vi "test4-ArgumentCanBeTakenToTargetModule.vi"(8 "error in (no error)":errorcluster, 11 "TestCase in":refnum<class "testcase-CSMArgument.lvclass">) -> (0 "error out":errorcluster, 3 "TestCase out":refnum<class "testcase-CSMArgument.lvclass">)   [LabVIEW 2017, in "testcase-CSMArgument.lvclass"]
uses:
  testcase-CSMArgument.lvclass
  a780a543-d55d-4312-9572-3fc81e4783fb.vi
  <vilib>/addons/_JKI Toolkits/VI Tester/TestCase.llb/TestCase.lvclass
  src/user.lib/_NEVSTOP/Communicable State Machine(CSM)/Communicable State Machine.lvlib
  CSM/CSM-Testcase.lvlib
  C:/Program Files (x86)/National Instruments/LabVIEW 2017/vi.lib/addons/_JKI Toolkits/VI Tester/TestCase.llb/TestCase.lvclass
panel:
  out "LoopCount":i32
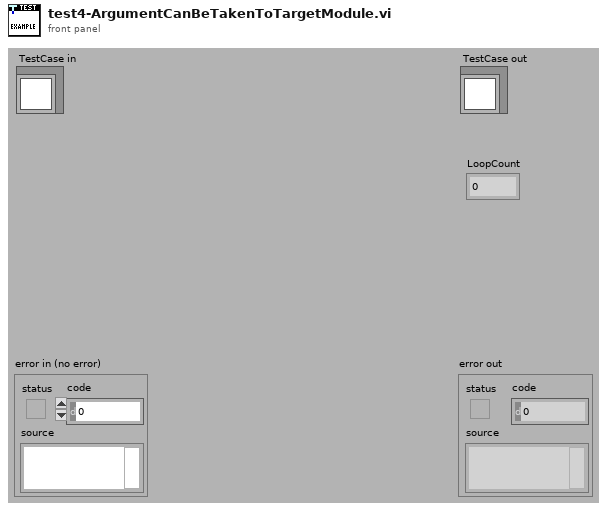
[diagram p1: front panel]
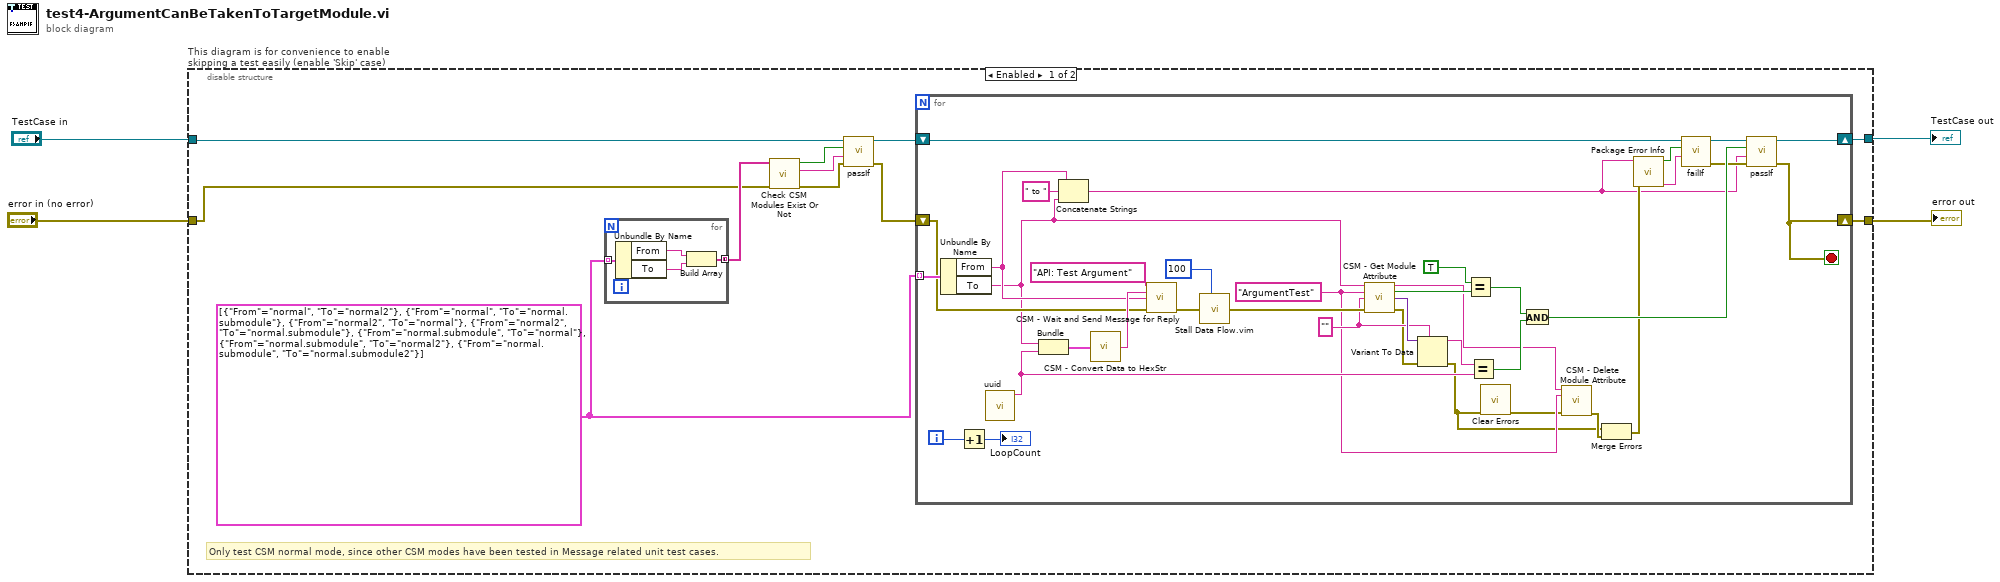
[diagram p0: block diagram]
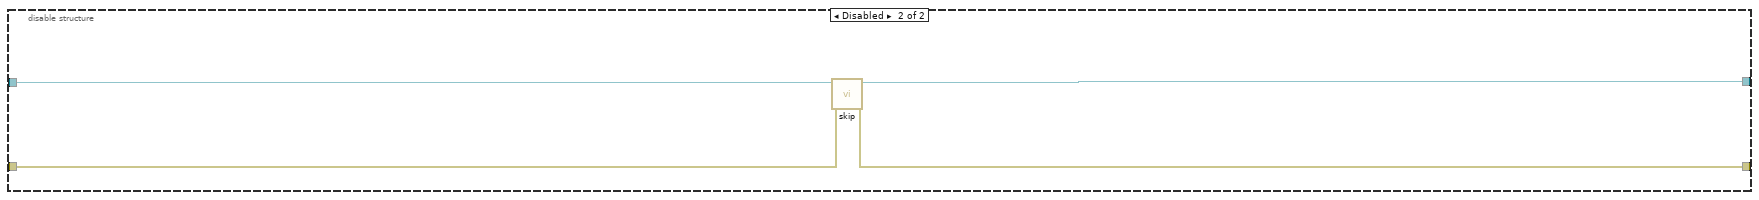
[diagram p2: hidden frame]
diagram:
  n1 = disable-structure "This diagram is for convenience to enable skipping a test easily (enable 'Skip' case)" shown="Enabled" {
    disable-tunnel: "TestCase in" -> [w8 w60]
    disable-tunnel: [w15 w58] -> w1
    disable-tunnel: [w14 w59] -> w3
    disable-tunnel: "error in (no error)" -> [w6 w57]
    frame Enabled {
      w9 = cluster{"From":string, "To":string}[] [{"From"="normal", "To"="normal2"}, {"From"="normal", "To"="normal.submodule"}, {"From"="normal2", "To"="normal"}, {"From"="normal2", "To"="normal.submodule"}, {"From"="normal.submodule", "To"="normal"}, {"From"="normal.submodule", "To"="normal2"}, {"From"="normal.submodule", "To"="normal.submodule2"}]
      # "Only test CSM normal mode, since other CSM modes have been tested in Message related unit test cases."
      n2 = for {
        tunnel: w9 -> [w19] mode=indexing
        tunnel: [w16] -> w12 mode=concatenating
        n3 = Unbundle By Name(w19) -> ("From"=w18:string, "To"=w17:string)
        n4 = Build Array(w18, w17) -> (w16:string[])
      }
      n5 = call "Check CSM Modules Exist Or Not.vi"("error in"=w6, "CSM names in"=w12) -> ("error out"=w10:errorcluster, "Debug string"=w11:string, "All Modules Exist?"=w13:bool)  [unwired: 7 in]
      n6 = call-dynamic "passIf.vi"("error in (no error)"=w10, "message (\"\")"=w11, "pass"=w13, "TestCase in"=w8) -> ("error out"=w5:errorcluster, "TestCase out"=w7:refnum<class "testcase-CSMArgument.lvclass">)  [unwired: 6 in]
      n7 = for {
        tunnel: w9 -> [w56] mode=indexing
        shift-right: [w42] -> w15
        shift-left: w7 -> [w26]
        shift-right: [w41] -> w14
        shift-left: w5 -> [w33]
        i -> [w40]
        stop <- w41 stop-if-true
        w46 = ""
        w34 = "ArgumentTest" ("Attribute")
        n8 = Unbundle By Name(w56) -> ("From"=w31:string, "To"=w29:string)
        n9 = Increment(x=w40) -> (x+1=→"LoopCount":i32)
        n10 = call "uuid.vi"() -> ("UUID"=w44:string)  [unwired: 11 in]
        n11 = Bundle("To"=w29, "UUID"=w44) -> (w51:cluster{"To":string, "UUID":string})  [unwired: 1 in]
        n12 = Concatenate Strings(w31, " to " ("string"), w29) -> (w20:string)
        n13 = call "CSM - Convert Data to HexStr.vi"("Variant"=w51) -> ("HEX String (0-9,A-F)"=w50:string)  [unwired: 8 in]
        n14 = call "CSM - Wait and Send Message for Reply.vi"("State"="API: Test Argument", "Arguments (\"\")"=w50, "Target Module"=w31, "Error In (No Error)"=w33) -> ("error out"=w54:errorcluster)  [unwired: 8 in, 3 out]
        n15 = call "Stall Data Flow.vim"("value in"=w54, "milliseconds to wait"=u32 100) -> ("value out"=w52:errorcluster)  [unwired: 1 out]
        n16 = call "CSM - Get Module Attribute.vi"("CSM Name"=w29, "Attribute"=w34, "Default Value (Empty Variant)"=w46, "Error In"=w52) -> ("CSM Name (Dup)"=w35:string, "Found"=w49:bool, "Value"=w47:variant, "error out"=w43:errorcluster)  [unwired: 7 in, 1 out]
        n17 = Variant To Data(error in=w43, type=w46, Variant=w47) -> (data=w45:string, error out=w22:errorcluster)
        n18 = Equal?(x=TRUE, y=w49) -> (x = y?=w38:bool)
        n19 = Equal?(x=w45, y=w44) -> (x = y?=w37:bool)
        n20 = call <vilib>:"Clear Errors.vi"("error in (no error)"=w22) -> ("error out"=w32:errorcluster)  [unwired: 5 in, 1 out]
        n21 = Compound Arithmetic op=AND(w38, w37) -> (w36:bool)
        n22 = call "CSM - Delete Module Attribute.vi"("CSM Name"=w35, "Attribute"=w34, "Error In"=w32) -> ("error out"=w23:errorcluster)  [unwired: 9 in, 3 out]
        n23 = Merge Errors(w22, w23) -> (w21:errorcluster)
        n24 = call "Package Error Info.vi"("error in"=w21, "String in"=w20) -> ("packed error info out"=w27:string, "error status"=w28:bool)  [unwired: 8 in]
        n25 = call-dynamic "failIf.vi"("message (\"\")"=w27, "fail"=w28, "TestCase in"=w26) -> ("error out"=w24:errorcluster, "TestCase out"=w25:refnum<class "testcase-CSMArgument.lvclass">)  [unwired: 7 in]
        n26 = call-dynamic "passIf.vi"("error in (no error)"=w24, "message (\"\")"=w20, "pass"=w36, "TestCase in"=w25) -> ("error out"=w41:errorcluster, "TestCase out"=w42:refnum<class "testcase-CSMArgument.lvclass">)  [unwired: 6 in]
      }
    }
    frame Disabled {
      # "skip test result while test is under development"
      n27 = call <vilib>:"skip.vi"("error in (no error)"=w57, "TestCase in"=w60) -> ("error out"=w59:errorcluster, "TestCase out"=w58:refnum<class "testcase-CSMArgument.lvclass">)  [unwired: 8 in]
    }
  }
  "error out" <- w3
  "TestCase out" <- w1
